vi "Convert to DI Module.vi"(8 "error in":errorcluster, 10 "slot ref in":T1 format="%.0x", 11 "module in":refnum<class "Module.lvclass">) -> (0 "error out":errorcluster, 2 "slot ref out":T1 format="%.0x", 3 "module out":refnum<class "Module.lvclass">)   [LabVIEW 2020, in "Scan Engine Scripting.lvlib"]
uses:
  Scan Engine Scripting.lvlib
  Modules/Module/Module.lvclass
  <vilib>/NI VeriStand/Custom Device API/Custom Device Item Ref.ctl
  Modules/Mode Classes/Digital Input Mode/Digital Input Mode.lvclass
  C:/jenkins/workspace/ercat-custom-device_release_20.4/Built/Scripting/Scan Engine/Modules/Mode Classes/Mode/Mode.lvclass
  b91a2346-f3dc-4342-9e9e-e10e54e4b359.vi
  <vilib>/NI VeriStand/Custom Device API/Custom Device API.lvlib
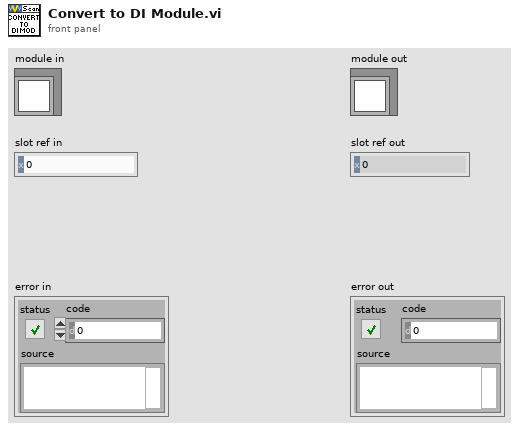
[diagram p1: front panel]
types:
  T1 = typedef "Custom Device API.lvlib/Custom Device Item Ref.ctl" = u64
  T2 = typedef "Scan Engine Scripting.lvlib/digital channel settings.ctl" = cluster{"name":string, "default value":bool}
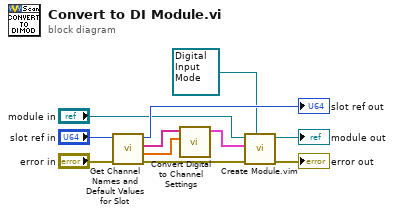
[diagram p0: block diagram]
diagram:
  n1 = call "Get Channel Names and Default Values for Slot.vi"("error in"="error in", "slot ref in"="slot ref in") -> ("error out"=w6:errorcluster, "channel default values"=w7:dbl[], "channel names"=w8:string[], "slot ref out"=→"slot ref out":T1)  [unwired: 6 in]
  n2 = call "Convert Digital to Channel Settings.vi"("channel default values"=w7, "channel names"=w8) -> ("channel settings"=w1:T2[])  [unwired: 9 in]
  n3 = call "Create Module.vim"("mode"=refnum<class "Digital Input Mode.lvclass"> refnum ("Scan Engine Scripting.lvlib:Digital Input Mode.lvclass"), "error in"=w6, "channel settings"=w1, "module in"="module in") -> ("error out"=→"error out":errorcluster, "module out"=→"module out":refnum<class "Module.lvclass">)  [unwired: 6 in]
